vi "File Exists.vi"(0 "Path In":path) -> (1 "Path Out":path, 2 "Append?":bool=TRUE)   [LabVIEW 2018]
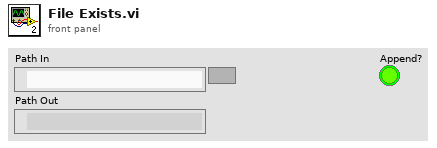
[diagram p1: front panel]
types:
  T1 = enum16{"Left Button", "Center Button", "Right Button", "Window Close"}
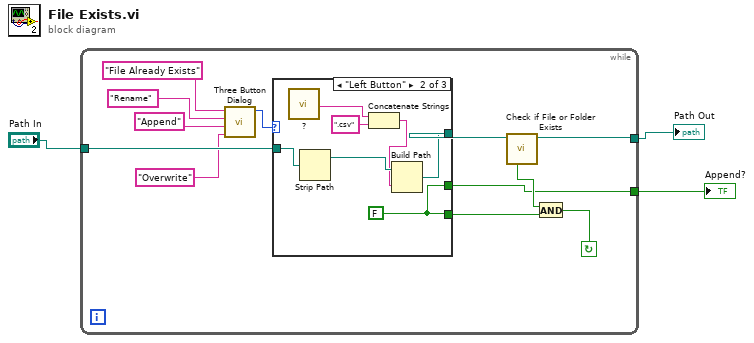
[diagram p0: block diagram]
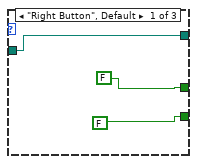
[diagram p2: hidden frame]
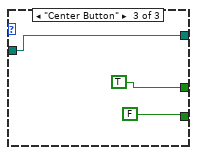
[diagram p3: hidden frame]
diagram:
  n1 = while {
    tunnel: [w15] -> w2
    tunnel: "Path In" -> [w13]
    tunnel: [w4] -> w1
    stop <- w10 continue-if-true
    n2 = call <vilib>:"Three Button Dialog.vi"("Right Button Text (\"Cancel\")"="Overwrite" ("T button name (\"OK\")"), "Center Button Text (\"No\")"="Append" ("F button name (\"Cancel\")"), "Left Button Text (\"Yes\")"="Rename" ("F button name (\"Cancel\")"), "message"="File Already Exists") -> ("Which Button?"=w8:T1)  [unwired: 7 in]
    n3 = case shown="\"Left Button\"" w8 {
      tunnel: w13 -> [w18 w25 w28]
      tunnel: [w18 w23 w28] -> w12
      tunnel: [FALSE w19 FALSE] -> w5
      tunnel: [FALSE w19 TRUE] -> w4
      frame "Right Button", Default {
      }
      frame "Left Button" {
        w19 = FALSE
        n4 = call "?"() -> ("Filename"=w22:string)  [unwired: 17 in, 2 out]
        n5 = Strip Path(path=w25) -> (stripped path=w24:path)  [unwired: 1 out]
        n6 = Concatenate Strings(w22, ".csv" ("string")) -> (w20:string)
        n7 = Build Path(base path=w24, name or relative path=w20) -> (appended path=w23:path)
      }
      frame "Center Button" {
      }
    }
    n8 = call <vilib>:"Check if File or Folder Exists.vi"("path"=w12) -> ("file or folder exists?"=w9:bool, "dup path"=w15:path)  [unwired: 8 in, 1 out]
    n9 = And(x=w9, y=w5) -> (x .and. y?=w10:bool)
  }
  "Path Out" <- w2
  "Append?" <- w1
